vi "progress bar ini.vi"(7 "text":string) -> ()   [LabVIEW 2017, in "util.lvlib"]
uses:
  util.lvlib
  progress bar GV.vi
panel:
  in  "Fehler (Eingang, kein Fehler)":errorcluster
  out "Fehler (Ausgang)":errorcluster
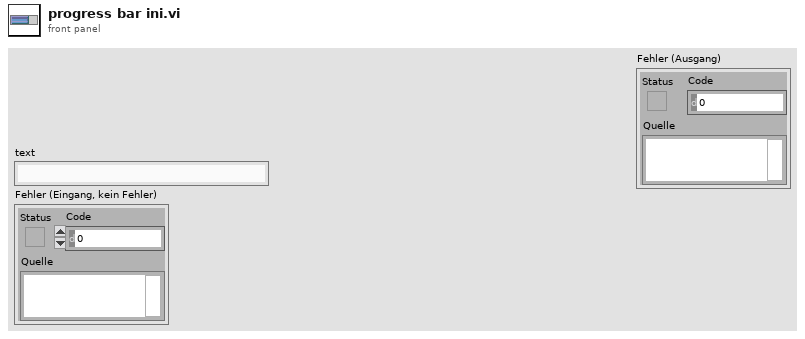
[diagram p1: front panel]
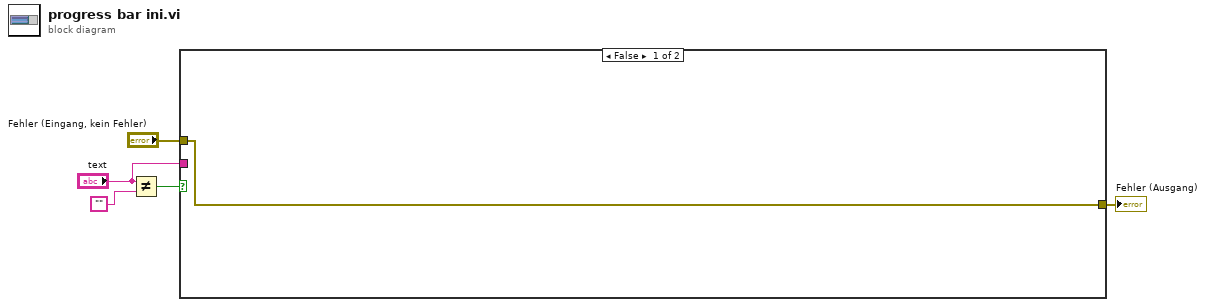
[diagram p0: block diagram]
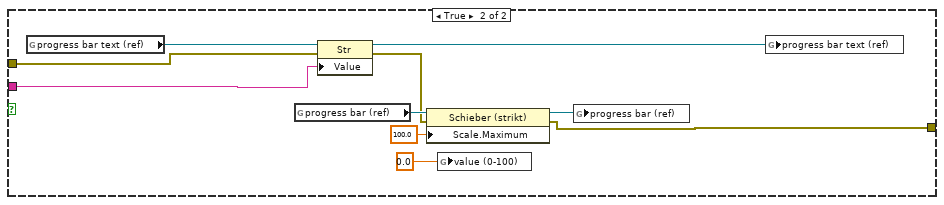
[diagram p2: hidden frame]
diagram:
  n1 = Not Equal?(x="text", y="") -> (x != y?=w3:bool)
  n2 = case shown="False" w3 {
    tunnel: "text" -> [_ w16]
    tunnel: [w6 w8] -> w2
    tunnel: "Fehler (Eingang, kein Fehler)" -> [w6 w7]
    frame False {
    }
    frame True {
      n3 = global read "progress bar GV.vi" "progress bar text (ref)"() -> (w10:refnum<vi>)
      n4 = global read "progress bar GV.vi" "progress bar (ref)"() -> (w14:refnum<vi>)
      n5 = property on="Eigenschaftsknoten" class="Str"(reference=w10, error in=w7, "Value"=w16) -> (reference out=w15:refnum<vi>, error out=w9:errorcluster)
      n6 = property on="Eigenschaftsknoten" class="Schieber (strikt)"(reference=w14, error in=w9, "Scale.Maximum"=100.0 ("Skala.Bereich:Maximum")) -> (reference out=w11:refnum<vi>, error out=w8:errorcluster)
      n7 = global write "progress bar GV.vi" "value (0-100)"(0.0 ("weight")) -> ()
      n8 = global write "progress bar GV.vi" "progress bar (ref)"(w11) -> ()
      n9 = global write "progress bar GV.vi" "progress bar text (ref)"(w15) -> ()
    }
  }
  "Fehler (Ausgang)" <- w2
